vi "Example.vi"() -> (0 "error out":errorcluster)   [LabVIEW 2022 SP3, in "PythonWrapper.lvlib"]
uses:
  PythonWrapper.lvlib
  PythonWrapper/PythonWrapper.lvclass
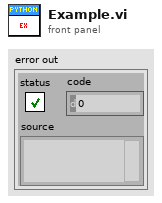
[diagram p1: front panel]
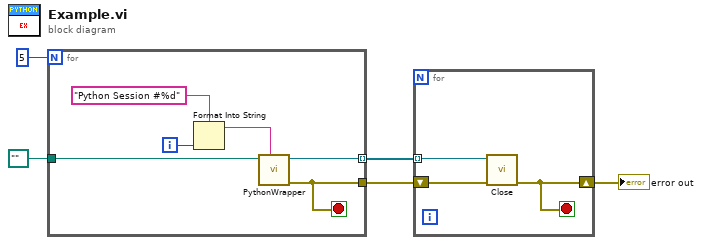
[diagram p0: block diagram]
diagram:
  n1 = for {
    N: 5 -> [_]
    tunnel: path "" ("ModulePath") -> [w11]
    tunnel: [w7] -> w3
    tunnel: [w6] -> w1 mode=indexing
    i -> [w10]
    stop <- w7 stop-if-true
    n2 = Format Into String(format string="Python Session #%d", w10) -> (resulting string=w9:string)  [unwired: 2 in, 1 out]
    n3 = call "PythonWrapper.vi"("SessionName"=w9, "ModulePath"=w11) -> ("error out"=w7:errorcluster, "PythonWrapper"=w6:refnum<class "PythonWrapper.lvclass">)  [unwired: 8 in]
  }
  n4 = for {
    tunnel: w1 -> [w12] mode=indexing
    shift-right: [w14] -> w2
    shift-left: w3 -> [w13]
    stop <- w14 stop-if-true
    n5 = call-dynamic "Close.vi"("error in (no error)"=w13, "PythonWrapper in"=w12) -> ("error out"=w14:errorcluster)  [unwired: 9 in]
  }
  "error out" <- w2
